vi "LS340_ConfigSerial.vi"(5 "error in":errorcluster, 8 "VISA":refnum<visa-resource-name>) -> (0 "error out":errorcluster, 2 "ID String":string, 3 "VISA Out":refnum<visa-resource-name>)   [LabVIEW 2012]
doc: "This VI passes the COM PORT to the VISA Config Serial VI and returns the instrument ID. \nIt reads ID back to test if the initialisation is successful. \n\nCall this before using any of the instrument driver VIs for this instrument.\n\n\nHARPS-N use"
uses:
  <vilib>/Instr/_visa.llb/VISA Configure Serial Port (Instr).vi
  <instrlib>/Lake Shore Cryotronics 218/Lake Shore Cryotronics 218.lvlib
panel:
  # "for HARPS-N use"
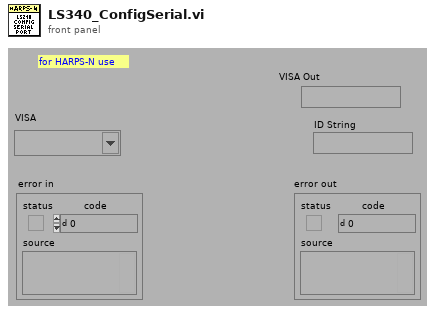
[diagram p1: front panel]
types:
  T1 = cluster{"Timeout Value (10000)":u32, "Baud Rate (57600)":enum16{"1200", "2400", "4800", "9600", "19200", "38400", "57600", "115200"}, "Flow Control (1:XON/XOFF)":enum16{"None", "XON / XOFF", "RTS / CTS", "DTR / DSR"}}
  T2 = enum16{"1200", "2400", "4800", "9600", "19200", "38400", "57600", "115200"}
  T3 = enum16{"None", "XON / XOFF", "RTS / CTS", "DTR / DSR"}
  T4 = cluster{"Status":bool, "Code":i32, "Source (VI Name)":string}
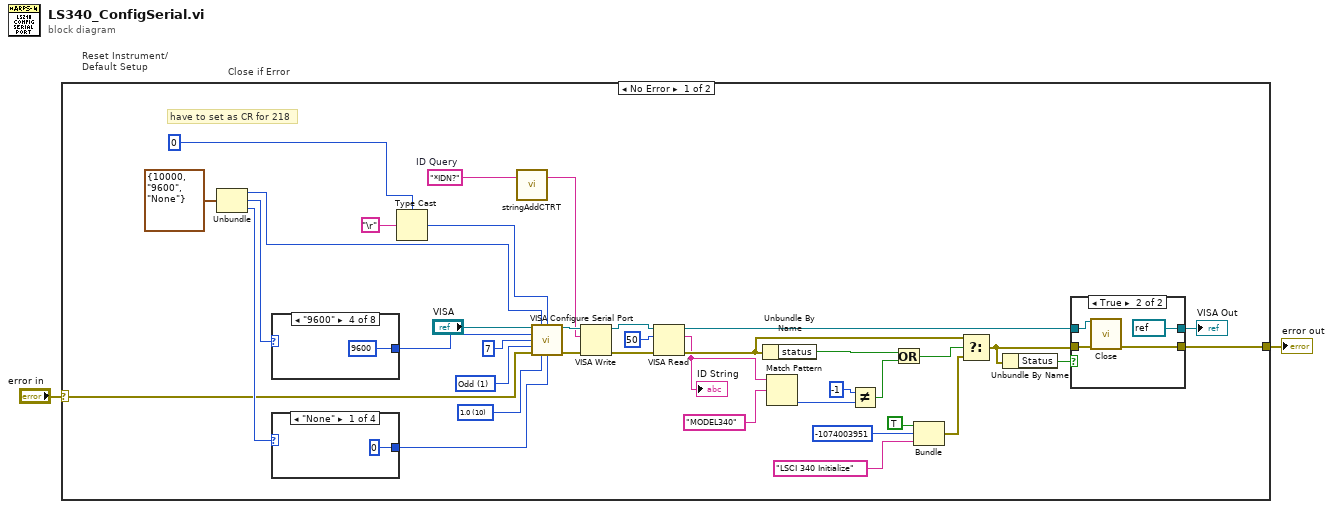
[diagram p0: block diagram]
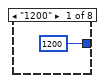
[diagram p3: hidden frame]
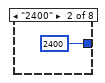
[diagram p4: hidden frame]
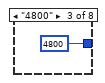
[diagram p5: hidden frame]
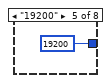
[diagram p6: hidden frame]
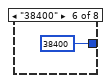
[diagram p7: hidden frame]
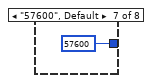
[diagram p8: hidden frame]
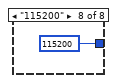
[diagram p9: hidden frame]
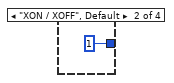
[diagram p10: hidden frame]
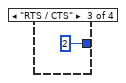
[diagram p11: hidden frame]
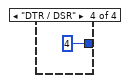
[diagram p12: hidden frame]
diagram:
  # "Close if Error"
  # "Reset Instrument/\nDefault Setup"
  n1 = case shown="No Error" "error in" {
    selector: "error in" -> [w28 w59]
    tunnel: [w9 w59] -> w1
    frame No Error {
      w4 = "*IDN?"  # ID Query
      w39 = u16 10 items=["1.0"=10, "1.5"=15, "2.0"=20] ("Serial Settings:Stop Bits")
      w38 = u16 1 items=["None", "Odd", "Even", "Mark", "Space"] ("Serial Settings:Serial Parity")
      # "have to set as CR for 218"
      n2 = Unbundle(T1 {"Timeout Value (10000)"=10000, "Baud Rate (57600)"=enum."9600", "Flow Control (1:XON/XOFF)"=enum."None"} ("Serial Port Configuration")) -> ("Timeout Value (10000)"=w36:u32, "Baud Rate (57600)"=w32:T2, "Flow Control (1:XON/XOFF)"=w33:T3)
      n3 = case shown="\"9600\"" w32 {
        tunnel: [u32 1200 u32 2400 u32 4800 u32 9600 u32 19200 u32 38400 u32 57600 u32 115200] -> w35
        frame "1200" {
        }
        frame "2400" {
        }
        frame "4800" {
        }
        frame "9600" {
        }
        frame "19200" {
        }
        frame "38400" {
        }
        frame "57600", Default {
        }
        frame "115200" {
        }
      }
      n4 = case shown="\"None\"" w33 {
        tunnel: [u16 0 u16 1 u16 2 u16 4] -> w34
        frame "None" {
        }
        frame "XON / XOFF", Default {
        }
        frame "RTS / CTS" {
        }
        frame "DTR / DSR" {
        }
      }
      n5 = Type Cast(type=u8 0, x="\r") -> (*(type *) &x=w29:u8)
      n6 = call "stringAddCTRT.vi"("string"=w4) -> ("strOut"=w3:string)  [unwired: 2 in]
      n7 = call-poly "VISA Configure Serial Port"("VISA resource name"="VISA", "timeout (10sec)"=w36, "termination char\n(0xA = '\\n' = LF)"=w29, "baud rate (9600)"=w35, "data bits (8)"=u16 7 ("Serial Settings:Serial Data Bits"), "parity (0:none)"=w38, "error in (no error)"=w28, "stop bits (10: 1 bit)"=w39, "flow control (0:none)"=w34) -> ("VISA resource name out"=w8:refnum<visa-resource-name>, "error out"=w12:errorcluster)  [unwired: 5 in]
      n8 = VISA Write(VISA resource name=w8, write buffer=w3, error in (no error)=w12) -> (VISA resource name out=w16:refnum<visa-resource-name>, error out=w18:errorcluster)  [unwired: 1 out]
      n9 = VISA Read(VISA resource name=w16, byte count=u32 50, error in (no error)=w18) -> (VISA resource name out=w7:refnum<visa-resource-name>, read buffer=w15:string, error out=w17:errorcluster)  [unwired: 1 out]
      "ID String" <- w15
      n10 = Unbundle By Name(w17) -> ("status"=w20:bool)
      n11 = Match Pattern(string=w15, regular expression="MODEL340") -> (offset past match=w23:i32)  [unwired: 1 in, 3 out]
      n12 = Not Equal?(x=-1, y=w23) -> (x != y?=w14:bool)
      n13 = Or(x=w20, y=w14) -> (x .or. y?=w19:bool)
      n14 = Bundle("Status"=TRUE, "Code"=-1074003951, "Source (VI Name)"="LSCI 340 Initialize") -> (w25:T4)  [unwired: 1 in]
      n15 = Select(t=w17, s=w19, f=w25) -> (s? t:f=w10:T4)
      n16 = Unbundle By Name(w10) -> ("Status"=w6:bool)
      n17 = case shown="True" w6 {
        tunnel: [w41 refnum<visa-resource-name> refnum ("VISA resource name out")] -> w11
        tunnel: [w42 w46] -> w9
        tunnel: w10 -> [w42 w44]
        tunnel: w7 -> [w41 w43]
        frame False {
        }
        frame True {
          n18 = call <instrlib>:"Close.vi"("VISA resource name"=w43, "error in (no error)"=w44) -> ("error out"=w46:errorcluster)  [unwired: 13 in]
        }
      }
      "VISA Out" <- w11
    }
    frame Error {
    }
  }
  "error out" <- w1
